vi "Variable_12kW_1kW.vi"() -> ()   [LabVIEW 2020]
panel:
  out "Voltage (V)":dbl
  in  "Power Supply":bool
  out "B":bool
  out "Y":bool
  out "R":bool
  out "No. of Resistors Used":i32
  out "Load (kW)":dbl
  out "Current (A)":dbl format="%.4f"
  in  "Load Selection":enum32{"1 kW", "12 kW"}(tab)
  in  "Step Type 1":enum32{"Variable Steps", "Equal Steps"}(tab)
  in  "Step_6\n250W":bool
  in  "Step_5\n250W":bool
  in  "Step_4\n200W":bool
  in  "Step_3\n150W":bool
  in  "Step_2\n100W":bool
  in  "Step_1\n50W":bool
  out "Step 1\nIndicator 6":bool
  out "Step 2\nIndicator 6":bool
  out "Step 3\nIndicator 5":bool
  out "Step 5\nIndicator 3":bool
  out "Step 6\nIndicator 3":bool
  out "Step 4\nIndicator 4":bool
  in  "1 equal steps":enum32{"2 Steps", "4 Steps"}(tab)
  out "Step 2\nIndicator 7":bool
  out "Step 1\nIndicator 7":bool
  in  "Step_1\n500W":bool
  in  "Step_2\n500W":bool
  out "Step 4\nIndicator 5":bool
  out "Step 3\nIndicator 6":bool
  out "Step 2\nIndicator 8":bool
  out "Step 1\nIndicator 8":bool
  in  "Step_1\n250W":bool
  in  "Step_2\n250W":bool
  in  "Step_3\n250W":bool
  in  "Step_4\n250W":bool
  in  "Master Switch 2":bool
  in  "Master Switch":bool
  in  "Step Type 12":enum32{"Variable Steps", "Equal Steps"}(tab)
  out "Step 7\nIndicator":bool
  out "Step 4\nIndicator":bool
  out "Step 10\nIndicator":bool
  out "Step 9\nIndicator":bool
  out "Step 8\nIndicator":bool
  out "Step 6\nIndicator":bool
  out "Step 5\nIndicator":bool
  out "Step 3\nIndicator":bool
  out "Step 2\nIndicator":bool
  out "Step 1\nIndicator":bool
  in  "Step 1\n250W":bool
  in  "Step 2\n250W":bool
  in  "Step 3\n500W":bool
  in  "Step 4\n1000W":bool
  in  "Step 5\n1000W":bool
  in  "Step 6\n1000W":bool
  in  "Step 7\n2000W":bool
  in  "Step 8\n2000W":bool
  in  "Step 9\n2000W":bool
  in  "Step 10\n2000W":bool
  in  "No. of Equal Steps":T1(tab)
  in  "Step 2\n6000W":bool
  in  "Step 1\n6000W":bool
  out "Step 1\nIndicator 3":bool
  out "Step 2\nIndicator 3":bool
  in  "Step 3\n4000W":bool
  in  "Step 2\n4000W":bool
  in  "Step 1\n4000W":bool
  out "Step 1\nIndicator 4":bool
  out "Step 2\nIndicator 4":bool
  out "Step 3\nIndicator 3":bool
  in  "Step 4\n3000W":bool
  in  "Step 3\n3000W":bool
  in  "Step 2\n3000W":bool
  in  "Step 1\n3000W":bool
  out "Step 1\nIndicator 5":bool
  out "Step 2\nIndicator 5":bool
  out "Step 3\nIndicator 4":bool
  out "Step 4\nIndicator 3":bool
  in  "Step 6\n2000W":bool
  in  "Step 5\n2000W":bool
  in  "Step 4\n2000W":bool
  in  "Step 3\n2000W":bool
  in  "Step 2\n2000W":bool
  in  "Step 1\n2000W":bool
  out "Step 1\nIndicator 2":bool
  out "Step 2\nIndicator 2":bool
  out "Step 3\nIndicator 2":bool
  out "Step 5\nIndicator 2":bool
  out "Step 6\nIndicator 2":bool
  out "Step 4\nIndicator 2":bool
  # "Three Phase Variable Resistive Load Bank with 1kW and 12kW Loads"
  # "All resistors are connected in 3 phase star formation"
  # "3 Phase Voltage Indicator"
  # "Select Value of Load"
  # "Resistors in Use"
  # "Resistors in Use"
  # "Resistors in Use"
  # "Resistors in Use"
  # "Resistors in Use"
  # "Resistors in Use"
  # "Resistors in Use"
  # "Resistors in Use"
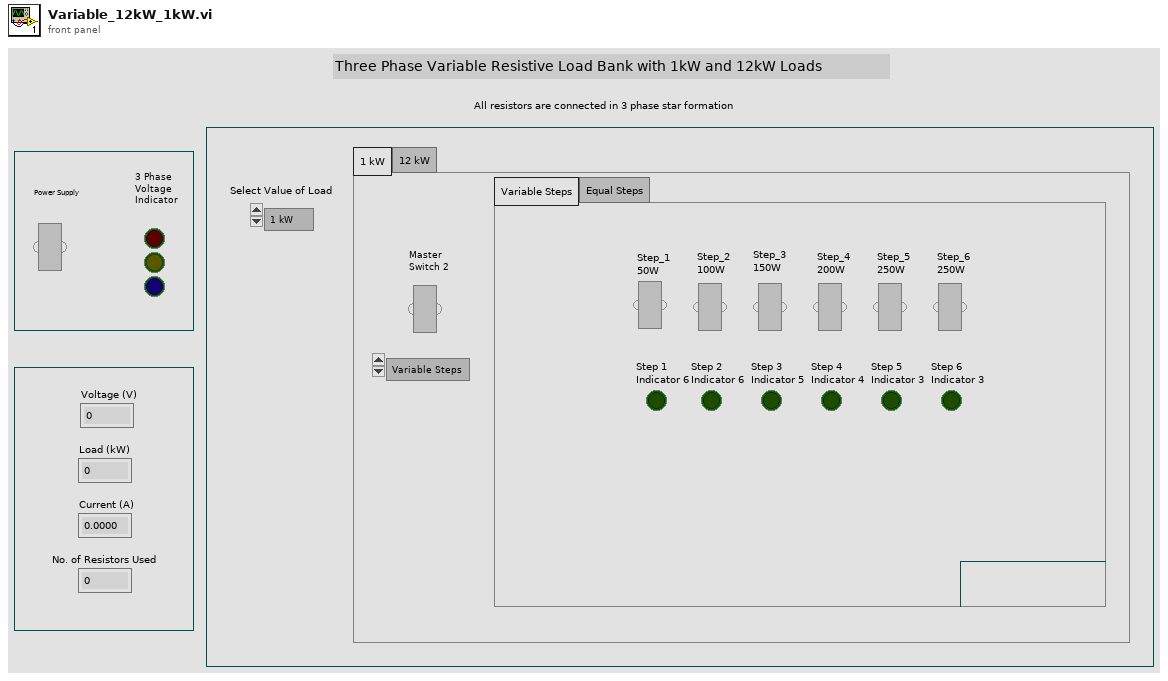
[diagram p1: front panel]
types:
  T1 = enum32{"2 Steps", "3 Steps", "4 Steps", "6 Steps"}
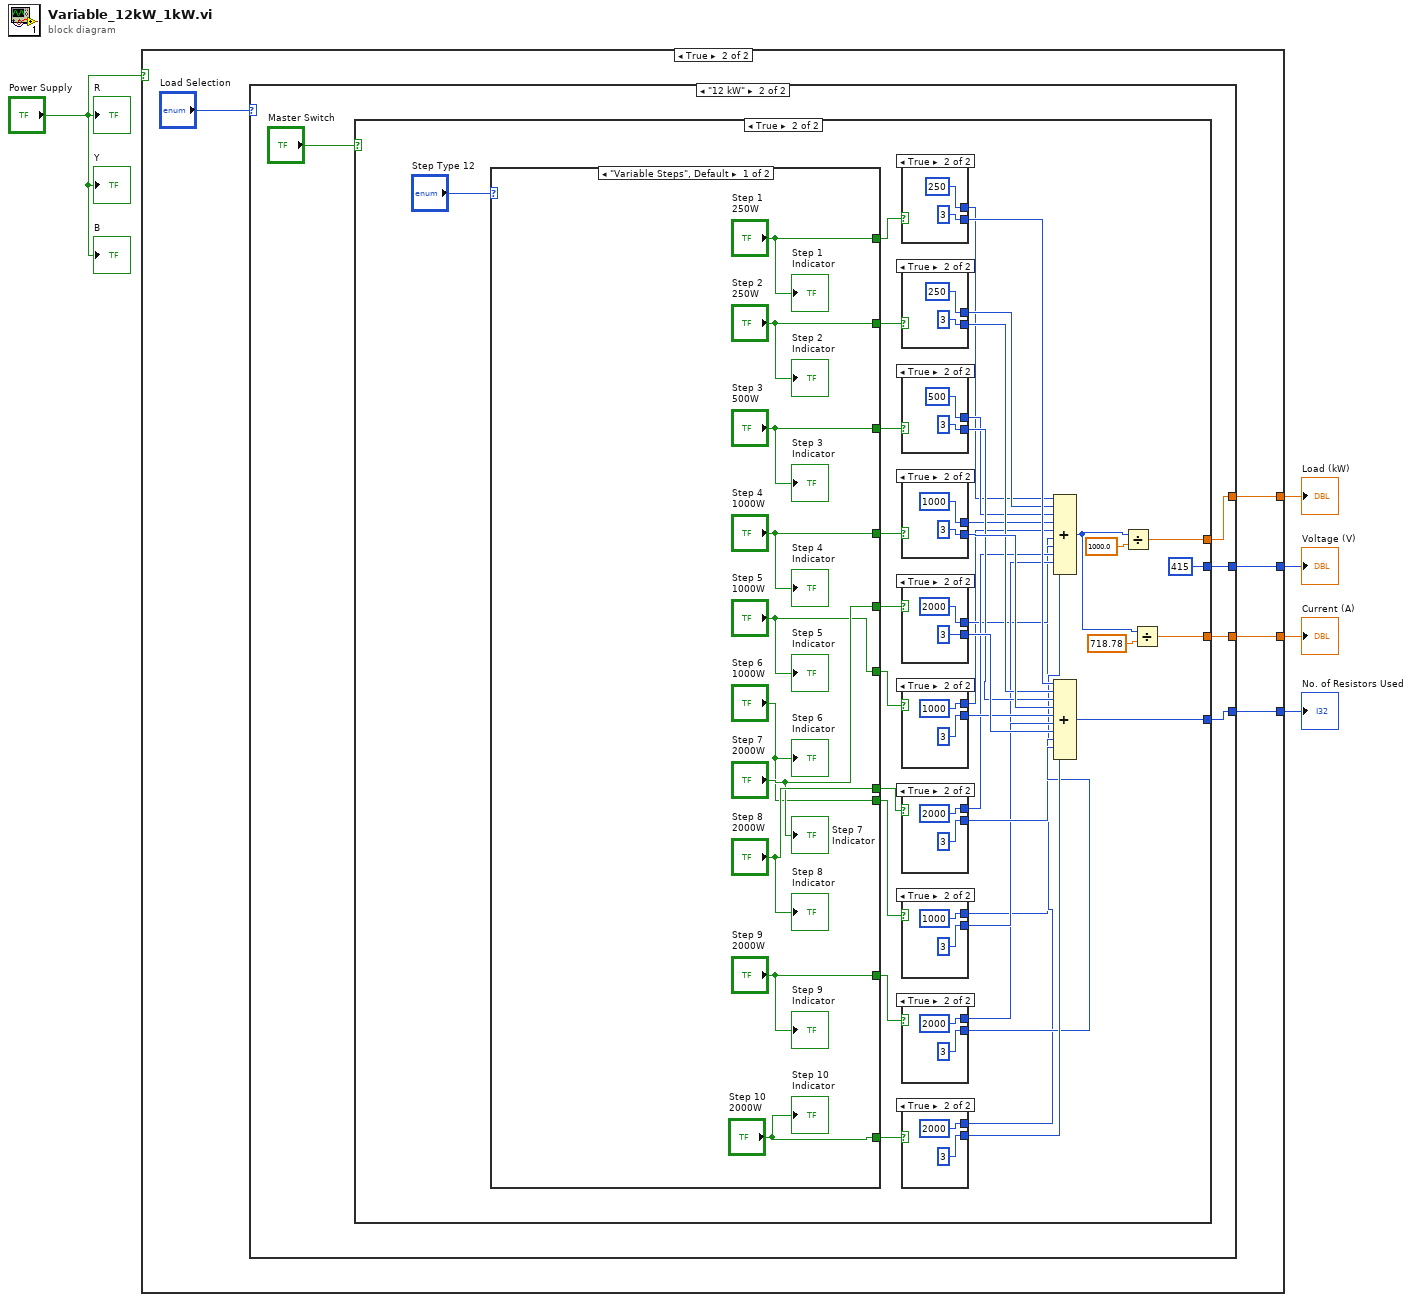
[diagram p0: block diagram]
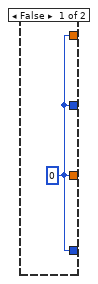
[diagram p2: hidden frame]
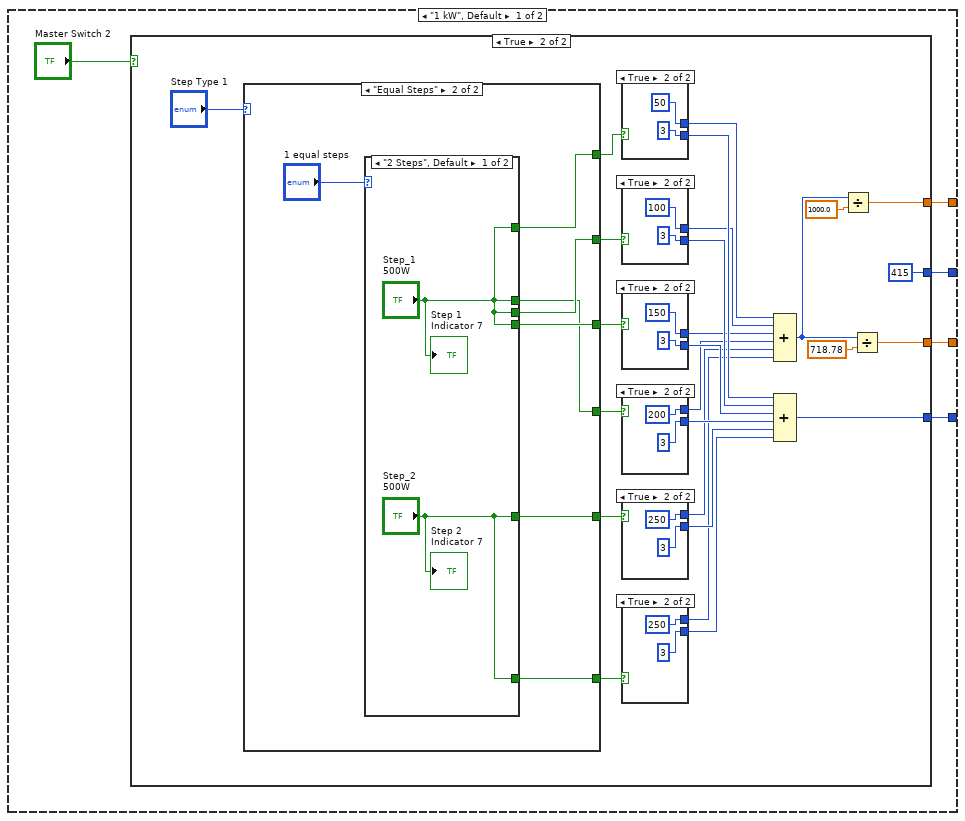
[diagram p3: hidden frame]
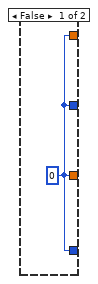
[diagram p4: hidden frame]
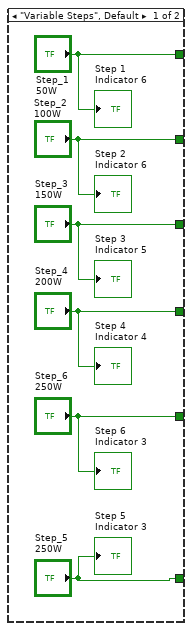
[diagram p5: hidden frame]
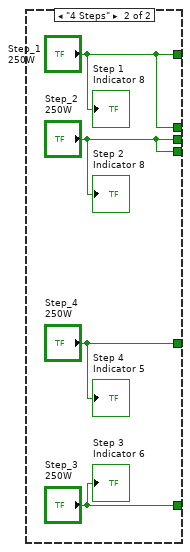
[diagram p6: hidden frame]
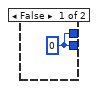
[diagram p7: hidden frame]
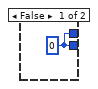
[diagram p8: hidden frame]
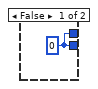
[diagram p9: hidden frame]
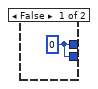
[diagram p10: hidden frame]
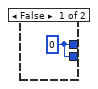
[diagram p11: hidden frame]
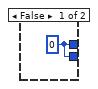
[diagram p12: hidden frame]
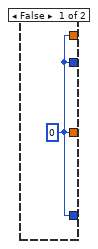
[diagram p13: hidden frame]
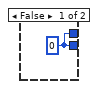
[diagram p14: hidden frame]
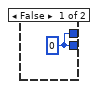
[diagram p15: hidden frame]
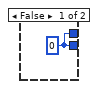
[diagram p16: hidden frame]
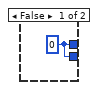
[diagram p17: hidden frame]
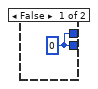
[diagram p18: hidden frame]
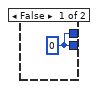
[diagram p19: hidden frame]
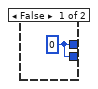
[diagram p20: hidden frame]
diagram:
  n1 = case shown="True" "Power Supply" {
    tunnel: [w6 w7] -> w5
    tunnel: [w6 w9] -> w3
    tunnel: [w6 w10] -> w4
    tunnel: [w6 w8] -> w1
    frame False {
      w6 = 0
    }
    frame True {
      n2 = case shown="\"12 kW\"" "Load Selection" {
        tunnel: [w12 w84] -> w10
        tunnel: [w13 w83] -> w9
        tunnel: [w15 w82] -> w7
        tunnel: [w14 w81] -> w8
        frame "1 kW", Default {
          n3 = case shown="True" "Master Switch 2" {
            tunnel: [w17 w30] -> w15
            tunnel: [w17 415] -> w14
            tunnel: [w17 w28] -> w13
            tunnel: [w17 w27] -> w12
            frame False {
              w17 = 0
            }
            frame True {
              n4 = case shown="\"Equal Steps\"" "Step Type 1" {
                tunnel: ["Step_1\n50W" w55] -> w23
                tunnel: ["Step_2\n100W" w54] -> w22
                tunnel: ["Step_3\n150W" w53] -> w21
                tunnel: ["Step_4\n200W" w52] -> w20
                tunnel: ["Step_5\n250W" w51] -> w19
                tunnel: ["Step_6\n250W" w50] -> w18
                frame "Variable Steps", Default {
                  "Step 1\nIndicator 6" <- "Step_1\n50W"
                  "Step 2\nIndicator 6" <- "Step_2\n100W"
                  "Step 3\nIndicator 5" <- "Step_3\n150W"
                  "Step 4\nIndicator 4" <- "Step_4\n200W"
                  "Step 5\nIndicator 3" <- "Step_5\n250W"
                  "Step 6\nIndicator 3" <- "Step_6\n250W"
                }
                frame "Equal Steps" {
                  n5 = case shown="\"2 Steps\", Default" "1 equal steps" {
                    tunnel: ["Step_1\n500W" "Step_1\n250W"] -> w55
                    tunnel: ["Step_1\n500W" "Step_2\n250W"] -> w54
                    tunnel: ["Step_1\n500W" "Step_2\n250W"] -> w53
                    tunnel: ["Step_1\n500W" "Step_1\n250W"] -> w52
                    tunnel: ["Step_2\n500W" "Step_3\n250W"] -> w51
                    tunnel: ["Step_2\n500W" "Step_4\n250W"] -> w50
                    frame "2 Steps", Default {
                      "Step 1\nIndicator 7" <- "Step_1\n500W"
                      "Step 2\nIndicator 7" <- "Step_2\n500W"
                    }
                    frame "4 Steps" {
                      "Step 1\nIndicator 8" <- "Step_1\n250W"
                      "Step 2\nIndicator 8" <- "Step_2\n250W"
                      "Step 3\nIndicator 6" <- "Step_3\n250W"
                      "Step 4\nIndicator 5" <- "Step_4\n250W"
                    }
                  }
                }
              }
              n6 = case shown="True" w23 {
                tunnel: [w78 50] -> w32
                tunnel: [w78 3] -> w37
                frame False {
                  w78 = 0
                }
                frame True {
                }
              }
              n7 = case shown="True" w22 {
                tunnel: [w75 100] -> w33
                tunnel: [w75 3] -> w38
                frame False {
                  w75 = 0
                }
                frame True {
                }
              }
              n8 = case shown="True" w21 {
                tunnel: [w72 150] -> w34
                tunnel: [w72 3] -> w39
                frame False {
                  w72 = 0
                }
                frame True {
                }
              }
              n9 = case shown="True" w20 {
                tunnel: [w69 200] -> w35
                tunnel: [w69 3] -> w40
                frame False {
                  w69 = 0
                }
                frame True {
                }
              }
              n10 = case shown="True" w18 {
                tunnel: [w66 250] -> w36
                tunnel: [w66 3] -> w41
                frame False {
                  w66 = 0
                }
                frame True {
                }
              }
              n11 = case shown="True" w19 {
                tunnel: [w63 250] -> w25
                tunnel: [w63 3] -> w26
                frame False {
                  w63 = 0
                }
                frame True {
                }
              }
              n12 = Compound Arithmetic op=ADD(w32, w33, w34, w35, w36, w25) -> (w31:i32)
              n13 = Compound Arithmetic op=ADD(w37, w38, w39, w40, w41, w26) -> (w27:i32)
              n14 = Divide(x=w31, y=1000.0) -> (x/y=w30:dbl)
              n15 = Divide(x=w31, y=718.78) -> (x/y=w28:dbl)
            }
          }
        }
        frame "12 kW" {
          n16 = case shown="True" "Master Switch" {
            tunnel: [w86 w91] -> w84
            tunnel: [w86 w87] -> w83
            tunnel: [w86 w88] -> w82
            tunnel: [w86 415] -> w81
            frame False {
              w86 = 0
            }
            frame True {
              n17 = case shown="\"Variable Steps\", Default" "Step Type 12" {
                tunnel: ["Step 10\n2000W" w165] -> w101
                tunnel: ["Step 9\n2000W" w166] -> w100
                tunnel: ["Step 8\n2000W" w167] -> w99
                tunnel: ["Step 7\n2000W" w168] -> w98
                tunnel: ["Step 6\n1000W" w169] -> w97
                tunnel: ["Step 5\n1000W" w170] -> w96
                tunnel: ["Step 4\n1000W" w171] -> w95
                tunnel: ["Step 3\n500W" w172] -> w94
                tunnel: ["Step 2\n250W" w173] -> w93
                tunnel: ["Step 1\n250W" w174] -> w92
                frame "Variable Steps", Default {
                  "Step 1\nIndicator" <- "Step 1\n250W"
                  "Step 4\nIndicator" <- "Step 4\n1000W"
                  "Step 7\nIndicator" <- "Step 7\n2000W"
                  "Step 2\nIndicator" <- "Step 2\n250W"
                  "Step 3\nIndicator" <- "Step 3\n500W"
                  "Step 5\nIndicator" <- "Step 5\n1000W"
                  "Step 8\nIndicator" <- "Step 8\n2000W"
                  "Step 9\nIndicator" <- "Step 9\n2000W"
                  "Step 10\nIndicator" <- "Step 10\n2000W"
                  "Step 6\nIndicator" <- "Step 6\n1000W"
                }
                frame "Equal Steps" {
                  n18 = case shown="\"2 Steps\", Default" "No. of Equal Steps" {
                    tunnel: ["Step 1\n6000W" "Step 1\n4000W" "Step 1\n3000W" "Step 1\n2000W"] -> w174
                    tunnel: ["Step 1\n6000W" "Step 1\n4000W" "Step 1\n3000W" "Step 1\n2000W"] -> w173
                    tunnel: ["Step 1\n6000W" "Step 1\n4000W" "Step 1\n3000W" "Step 1\n2000W"] -> w172
                    tunnel: ["Step 1\n6000W" "Step 1\n4000W" "Step 2\n3000W" "Step 1\n2000W"] -> w171
                    tunnel: ["Step 1\n6000W" "Step 1\n4000W" "Step 3\n3000W" "Step 2\n2000W"] -> w170
                    tunnel: ["Step 1\n6000W" "Step 1\n4000W" "Step 4\n3000W" "Step 2\n2000W"] -> w169
                    tunnel: ["Step 1\n6000W" "Step 2\n4000W" "Step 1\n3000W" "Step 3\n2000W"] -> w168
                    tunnel: ["Step 2\n6000W" "Step 2\n4000W" "Step 2\n3000W" "Step 4\n2000W"] -> w167
                    tunnel: ["Step 2\n6000W" "Step 3\n4000W" "Step 3\n3000W" "Step 5\n2000W"] -> w166
                    tunnel: ["Step 2\n6000W" "Step 3\n4000W" "Step 4\n3000W" "Step 6\n2000W"] -> w165
                    frame "2 Steps", Default {
                      "Step 2\nIndicator 3" <- "Step 2\n6000W"
                      "Step 1\nIndicator 3" <- "Step 1\n6000W"
                    }
                    frame "3 Steps" {
                      "Step 1\nIndicator 4" <- "Step 1\n4000W"
                      "Step 3\nIndicator 3" <- "Step 3\n4000W"
                      "Step 2\nIndicator 4" <- "Step 2\n4000W"
                    }
                    frame "4 Steps" {
                      "Step 3\nIndicator 4" <- "Step 3\n3000W"
                      "Step 2\nIndicator 5" <- "Step 2\n3000W"
                      "Step 1\nIndicator 5" <- "Step 1\n3000W"
                      "Step 4\nIndicator 3" <- "Step 4\n3000W"
                    }
                    frame "6 Steps" {
                      "Step 1\nIndicator 2" <- "Step 1\n2000W"
                      "Step 6\nIndicator 2" <- "Step 6\n2000W"
                      "Step 5\nIndicator 2" <- "Step 5\n2000W"
                      "Step 2\nIndicator 2" <- "Step 2\n2000W"
                      "Step 3\nIndicator 2" <- "Step 3\n2000W"
                      "Step 4\nIndicator 2" <- "Step 4\n2000W"
                    }
                  }
                }
              }
              n19 = case shown="True" w92 {
                tunnel: [w152 250] -> w102
                tunnel: [w152 3] -> w112
                frame False {
                  w152 = 0
                }
                frame True {
                }
              }
              n20 = case shown="True" w93 {
                tunnel: [w149 250] -> w103
                tunnel: [w149 3] -> w113
                frame False {
                  w149 = 0
                }
                frame True {
                }
              }
              n21 = case shown="True" w94 {
                tunnel: [w146 500] -> w104
                tunnel: [w146 3] -> w114
                frame False {
                  w146 = 0
                }
                frame True {
                }
              }
              n22 = case shown="True" w95 {
                tunnel: [w143 1000] -> w105
                tunnel: [w143 3] -> w115
                frame False {
                  w143 = 0
                }
                frame True {
                }
              }
              n23 = case shown="True" w98 {
                tunnel: [w134 2000] -> w108
                tunnel: [w134 3] -> w118
                frame False {
                  w134 = 0
                }
                frame True {
                }
              }
              n24 = case shown="True" w96 {
                tunnel: [w140 1000] -> w106
                tunnel: [w140 3] -> w116
                frame False {
                  w140 = 0
                }
                frame True {
                }
              }
              n25 = case shown="True" w99 {
                tunnel: [w131 2000] -> w109
                tunnel: [w131 3] -> w119
                frame False {
                  w131 = 0
                }
                frame True {
                }
              }
              n26 = case shown="True" w97 {
                tunnel: [w137 1000] -> w107
                tunnel: [w137 3] -> w117
                frame False {
                  w137 = 0
                }
                frame True {
                }
              }
              n27 = case shown="True" w100 {
                tunnel: [w128 2000] -> w110
                tunnel: [w128 3] -> w120
                frame False {
                  w128 = 0
                }
                frame True {
                }
              }
              n28 = case shown="True" w101 {
                tunnel: [w125 2000] -> w111
                tunnel: [w125 3] -> w121
                frame False {
                  w125 = 0
                }
                frame True {
                }
              }
              n29 = Compound Arithmetic op=ADD(w102, w103, w104, w105, w106, w107, w108, w109, w110, w111) -> (w90:i32)
              n30 = Compound Arithmetic op=ADD(w112, w113, w114, w115, w116, w117, w118, w119, w120, w121) -> (w91:i32)
              n31 = Divide(x=w90, y=1000.0) -> (x/y=w88:dbl)
              n32 = Divide(x=w90, y=718.78) -> (x/y=w87:dbl)
            }
          }
        }
      }
    }
  }
  "Load (kW)" <- w5
  "Current (A)" <- w3
  "No. of Resistors Used" <- w4
  "Voltage (V)" <- w1
  "B" <- "Power Supply"
  "Y" <- "Power Supply"
  "R" <- "Power Supply"
